vi "Max Bin transfer.vi"() -> (0 "Time Out?":bool)   [LabVIEW 2014]
uses:
  <vilib>/rvi/Emulation/niFpgaEmulationIsFPGAContextNoSignature.vi
  <vilib>/rvi/DataTransferAndStorage/Container/Common/niFpgaContainerGetUniqueNameForEmu.vi
  <vilib>/rvi/Memory/Memory_Emulation/niFpgaMemoryEmulationCacheClearOnFirstRun.vi
  <vilib>/rvi/Memory/Memory_Emulation/nirvimemoryEmulationManagerCache_MakeExclusive.vi
  <vilib>/rvi/Memory/Memory_Emulation/niFpgaMemoryEmulationValidateCache.vi
  <vilib>/rvi/Memory/Memory_Emulation/nirvimemoryEmulationManagerCache_InsertValue.vi
  <vilib>/Utility/error.llb/Clear Errors.vi
  <vilib>/rvi/Memory/Memory_Emulation/nirvimemoryEmulationManagerCache_ReleaseExclusive.vi
  <vilib>/rvi/Memory/Memory_Emulation/nirvimemoryEmulationManagerCache_GetValue.vi
  <vilib>/rvi/Memory/Memory_Emulation/nirvimemoryEmulationManagerCache_SetValue.vi
  <vilib>/rvi/Emulation/niFpgaProcessEmulError.vi
  <vilib>/rvi/Emulation/niFpgaSctlEmulationGetInTimedLoop.vi
  <vilib>/rvi/interface/RandomDataEmulation/niFpgaRandomDataHandleErrors.vi
  <vilib>/rvi/DataTransferAndStorage/Container/XNode/niFpgaContainer.xnode
  <vilib>/rvi/DataTransferAndStorage/Register/Emulation/niFpgaRegisterEmulation.vi
  <vilib>/rvi/interface/RandomDataEmulation/nirviRandomDataFpgaReadWriteTemplate.vi
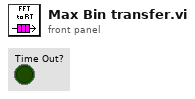
[diagram p1: front panel]
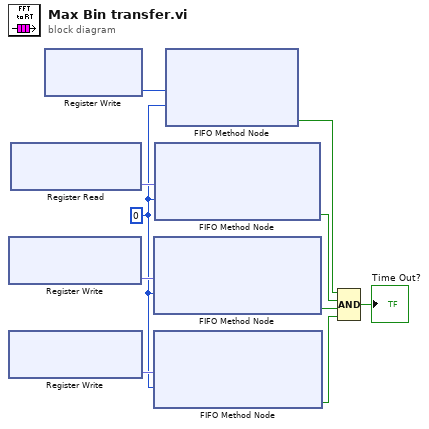
[diagram p0: block diagram]
diagram:
  w6 = 0 ("Timeout")
  n1 = xnode "Register Write"() -> ("Data"=w8:fxp<+,44,44>)  [unwired: 1 in, 1 out]
  n2 = xnode "Register Write"() -> ("Data"=w7:fxp<+,44,44>)  [unwired: 1 in, 1 out]
  n3 = xnode "Register Read"() -> ("Data"=w9:fxp<+,44,44>)  [unwired: 1 in, 1 out]
  n4 = xnode "Register Write"() -> ("Data"=w10:i32)  [unwired: 1 in, 1 out]
  n5 = xnode ("FIFO Method Node")("Element"=w8, "Timeout"=w6) -> ("Timed Out?"=w5:bool)  [unwired: 1 in, 1 out]
  n6 = xnode ("FIFO Method Node")("Element"=w7, "Timeout"=w6) -> ("Timed Out?"=w3:bool)  [unwired: 1 in, 1 out]
  n7 = xnode ("FIFO Method Node")("Element"=w9, "Timeout"=w6) -> ("Timed Out?"=w2:bool)  [unwired: 1 in, 1 out]
  n8 = xnode ("FIFO Method Node")("Element"=w10, "Timeout"=w6) -> ("Timed Out?"=w1:bool)  [unwired: 1 in, 1 out]
  n9 = Compound Arithmetic op=AND(w1, w2, w5, w3) -> (→"Time Out?":bool)
